vi "SetCol.vi"(4 "ModeCol Index":i32=2, 5 "Col Array Ref in":refnum<vi>, 6 "Cell Position":T1, 7 "Table History ref":refnum<vi>, 8 "error in (no error)":errorcluster, 9 "Table CtlRef In":refnum<vi>, 10 "SetTo":string, 11 "DigitalCol in":refnum<class "DigitalCol.lvclass">) -> (0 "error out":errorcluster, 1 "Table CtlRef Out":refnum<vi>, 2 "Num Rows":i32, 3 "DigitalCol out":refnum<class "DigitalCol.lvclass">)   [LabVIEW 2013, in "DigitalCol.lvclass"]
doc: "Set all rows of a column in the table to \"SetTo\" and check the digital coloring.\n(This VI was formerly called directly from a user click, and therefore defers panel updates inside.)"
uses:
  DigitalCol.lvclass
  <vilib>/Utility/miscctls.llb/LVRowAndColumnTypeDef.ctl
  TypeDefs/TableHistory.ctl
  TypeDefs/TableArray.ctl
  Column/Column.lvclass
  Column/Column.lvclass/Column.ctl
  Globals/DisabledColorGlobal.vi
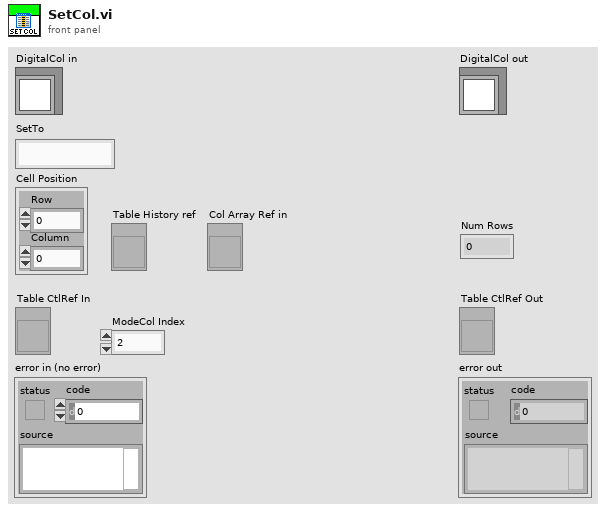
[diagram p1: front panel]
types:
  T1 = typedef "LVRowAndColumnTypeDef.ctl" = cluster{"Row":i32, "Column":i32}
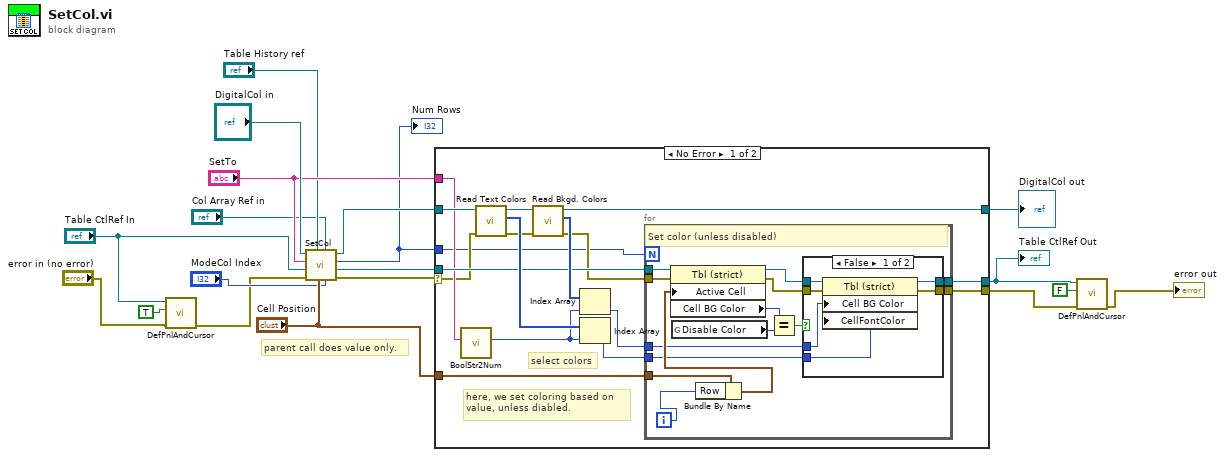
[diagram p0: block diagram]
diagram:
  # "parent call does value only."
  n1 = call "DefPnlAndCursor.vi"("error in (no error)"="error in (no error)", "DeferPanUpdts?"=TRUE ("Defer Panel Updates"), "Tbl Ctrl Refnum"="Table CtlRef In") -> ("error out"=w8:errorcluster)  [unwired: 8 in]
  n2 = call-parent "SetCol.vi"("ModeCol Index"="ModeCol Index", "Col Array Ref in"="Col Array Ref in", "Cell Position"="Cell Position", "Table History ref"="Table History ref", "error in (no error)"=w8, "Table CtlRef In"="Table CtlRef In", "SetTo"="SetTo", "Column in"="DigitalCol in") -> ("error out"=w13:errorcluster, "Table CtlRef Out"=w18:refnum<vi>, "Num Rows"=w12:i32, "Column out"=w17:refnum<class "DigitalCol.lvclass">)
  "Num Rows" <- w12
  n3 = case shown="No Error" w13 {
    selector: w13 -> [w21 w60]
    tunnel: w18 -> [w31 w61]
    tunnel: [w30 w61] -> w3
    tunnel: [w29 w60] -> w2
    tunnel: w17 -> [w26 w59]
    tunnel: [w25 w59] -> w16
    tunnel: "SetTo" -> [w23 _]
    tunnel: "Cell Position" -> [w22 _]
    tunnel: w12 -> [w20 _]
    frame No Error {
      # "here, we set coloring based on \nvalue, unless diabled."
      # "select colors"
      n4 = call "BoolStr2Num.vi"("Boolean string"=w23) -> ("number"=w33:i32)  [unwired: 10 in]
      n5 = call "Read Text Colors.vi"("error in (no error)"=w21, "Column in"=w26) -> ("error out"=w32:errorcluster, "Text Colors"=w35:u32[], "Column out"=w36:refnum<class "DigitalCol.lvclass">)  [unwired: 7 in]
      n6 = call "Read Bkgd. Colors.vi"("error in (no error)"=w32, "Column in"=w36) -> ("error out"=w24:errorcluster, "Bkgd. Colors"=w34:u32[], "Column out"=w25:refnum<class "DigitalCol.lvclass">)  [unwired: 7 in]
      n7 = Index Array(array=w34, index=w33) -> (element=w28:u32)
      n8 = Index Array(array=w35, index=w33) -> (element=w27:u32)
      n9 = for {
        N: w20 -> [_]
        tunnel: w28 -> [w39]
        tunnel: w27 -> [w38]
        tunnel: w24 -> [w45]
        tunnel: w31 -> [w47]
        tunnel: [w50] -> w30
        tunnel: w22 -> [w49]
        tunnel: [w48] -> w29
        i -> [w37]
        # "Set color (unless disabled)"
        n10 = global read "DisabledColorGlobal.vi" "Disable Color"() -> (w41:u32)
        n11 = Bundle By Name(cluster=w49, "Row"=w37) -> (w43:T1)
        n12 = property class="Tbl (strict)"(reference=w47, error in=w45, "Active Cell"=w43) -> (reference out=w46:refnum<vi>, error out=w44:errorcluster, "Cell BG Color"=w42:u32)
        n13 = Equal?(x=w42, y=w41) -> (x = y?=w40:bool)
        n14 = case shown="False" w40 {
          tunnel: [w56 w58] -> w50
          tunnel: [w55 w57] -> w48
          tunnel: w46 -> [w54 w58]
          tunnel: w44 -> [w53 w57]
          tunnel: w39 -> [w52 _]
          tunnel: w38 -> [w51 _]
          frame False {
            n15 = property class="Tbl (strict)"(reference=w54, error in=w53, "Cell BG Color"=w52, "CellFontColor"=w51) -> (reference out=w56:refnum<vi>, error out=w55:errorcluster)
          }
          frame True {
            # "leave disabled!"
          }
        }
      }
    }
    frame Error {
    }
  }
  "Table CtlRef Out" <- w3
  "DigitalCol out" <- w16
  n16 = call "DefPnlAndCursor.vi"("error in (no error)"=w2, "DeferPanUpdts?"=FALSE, "Tbl Ctrl Refnum"=w3) -> ("error out"=→"error out":errorcluster)  [unwired: 8 in]
